vi "Insert Key Value Pair (Nested Boolean).vi"(7 "key":string[](array[string]), 8 "error in (no error)":errorcluster, 10 "JSON Data in":bool, 11 "JSON Object in":refnum<class "JSON Helper.lvclass">) -> (0 "error out":errorcluster, 1 "replaced":bool, 3 "JSON Object Out":refnum<class "JSON Helper.lvclass">)   [LabVIEW 2016, in "JSON Helper.lvclass"]
uses:
  JSON Helper/JSON Helper.lvclass
  JSON Datatype/JSON Null.lvclass
  JSON Array/Replace Array Subset (Single).vi
  JSON Helper/To More Specific Type (Object).vi
  JSON Helper/To More Specific Type (Array).vi
  JSON Boolean/New JSON Boolean.vi
  Insert Key Value Pair (Single String).vi
  JSON Array/JSON Array.lvclass
  JSON Object.lvclass
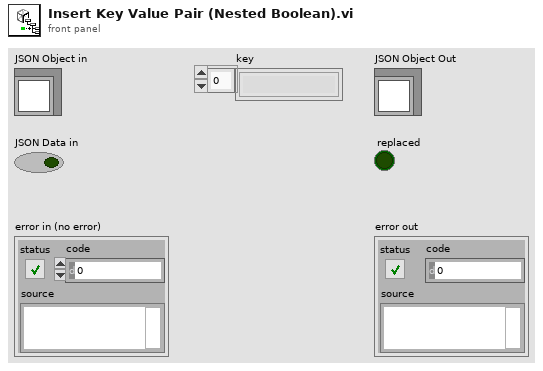
[diagram p1: front panel]
types:
  T1 = typedef "JSON Helper.lvclass/JSON Types.ctl" = enum16{"String", "Numeric", "Boolean", "NULL", "Object", "Array"}
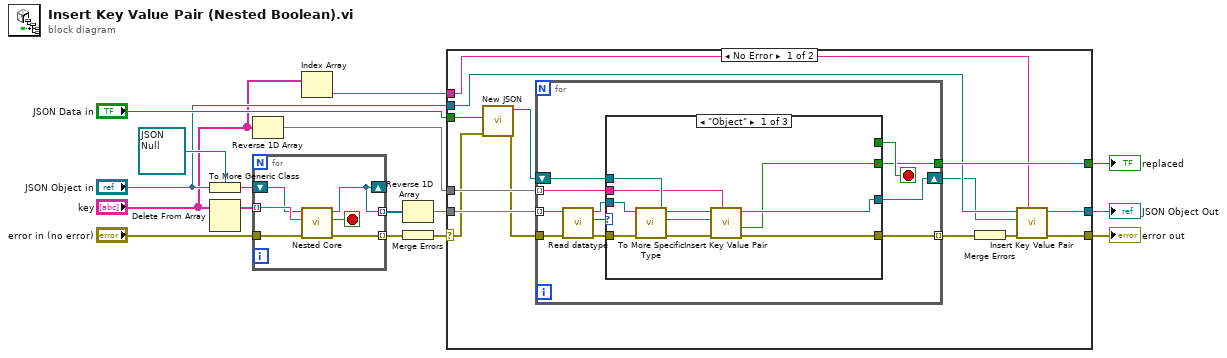
[diagram p0: block diagram]
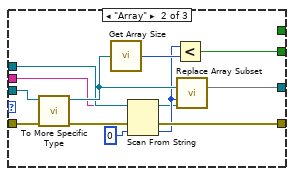
[diagram p2: hidden frame]
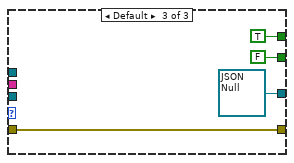
[diagram p3: hidden frame]
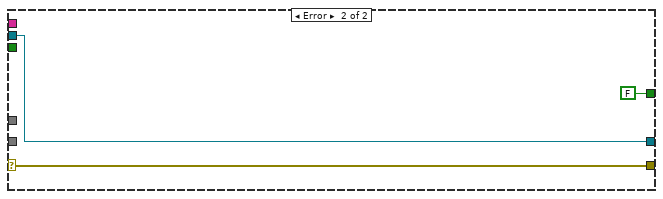
[diagram p4: hidden frame]
diagram:
  n1 = To More Generic Class(target class=refnum<class "JSON Null.lvclass"> refnum, reference="JSON Object in") -> (generic class reference=w8:refnum<class "JSON Null.lvclass">)
  n2 = Delete From Array(array="key") -> (array with subset deleted=w12:string[])  [unwired: 2 in, 1 out]
  n3 = Reverse 1D Array(array="key") -> (reversed array=w13:string[])
  n4 = for {
    tunnel: w12 -> [w22] mode=indexing
    shift-right: [w17] -> _
    shift-left: w8 -> [w21]
    tunnel: "error in (no error)" -> [w20]
    tunnel: [w19] -> w9 mode=indexing
    tunnel: [w17] -> w10 mode=indexing
    stop <- w18 stop-if-true
    n5 = call "Nested Core.vi"("error in (no error)"=w20, "key"=w22, "JSON in"=w21) -> ("error out"=w19:errorcluster, "stop?"=w18:bool, "JSON out"=w17:refnum<class "JSON Helper.lvclass">)  [unwired: 6 in]
  }
  n6 = Index Array(array="key") -> (element=w1:string)  [unwired: 1 in]
  n7 = Reverse 1D Array(array=w10) -> (reversed array=w14:refnum<class "JSON Helper.lvclass">[])
  n8 = Merge Errors(w9) -> (w11:errorcluster)
  n9 = case shown="No Error" w11 {
    selector: w11 -> [w24 w73]
    tunnel: [w36 FALSE ("replaced")] -> w16
    tunnel: "JSON Data in" -> [w26 _]
    tunnel: w14 -> [w35 _]
    tunnel: w13 -> [w34 _]
    tunnel: [w30 w75] -> w4
    tunnel: "JSON Object in" -> [w32 w75]
    tunnel: [w28 w73] -> w3
    tunnel: w1 -> [w27 _]
    frame No Error {
      n10 = call-poly "New JSON.vi"("error in (no error)"=w24, "value"=w26) -> ("error out"=w23:errorcluster, "JSON Boolean out"=w25:refnum<class "JSON Helper.lvclass">)  [unwired: 8 in]
      n11 = for {
        tunnel: w34 -> [w39] mode=indexing
        tunnel: w23 -> [w45]
        tunnel: [w44] -> w33 mode=indexing
        tunnel: [w41] -> w36
        tunnel: w35 -> [w40] mode=indexing
        shift-right: [w38] -> w31
        shift-left: w25 -> [w37]
        stop <- w42 stop-if-true
        n12 = call "Read datatype.vi"("error in (no error)"=w45, "JSON Datatype in"=w40) -> ("error out"=w43:errorcluster, "datatype"=w46:T1, "JSON Datatype out"=w47:refnum<class "JSON Helper.lvclass">)  [unwired: 7 in]
        n13 = case shown="\"Object\"" w46 {
          tunnel: w39 -> [w48 w57 _]
          tunnel: [w50 w59 refnum<class "JSON Null.lvclass"> refnum ("JSON Data")] -> w38
          tunnel: w47 -> [w55 w68 _]
          tunnel: [w52 w64 w70] -> w44
          tunnel: w43 -> [w54 w66 w70]
          tunnel: [_ _ TRUE] -> w42
          tunnel: [w49 w60 FALSE] -> w41
          tunnel: w37 -> [w51 w58 _]
          frame "Object" {
            n14 = call-poly "To More Specific Type.vi"("error in (no error)"=w54, "JSON Datatype in"=w55) -> ("error out"=w53:errorcluster, "JSON Datatype out"=w56:refnum<class "JSON Object.lvclass">)  [unwired: 8 in]
            n15 = call-poly "Insert Key Value Pair.vi"("key"=w48, "error in (no error)"=w53, "value"=w51, "JSON Object in"=w56) -> ("error out"=w52:errorcluster, "replaced"=w49:bool, "JSON Object out"=w50:refnum<class "JSON Helper.lvclass">)  [unwired: 5 in]
          }
          frame "Array" {
            n16 = call-poly "To More Specific Type.vi"("error in (no error)"=w66, "JSON Datatype in"=w68) -> ("error out"=w65:errorcluster, "JSON Datatype out"=w63:refnum<class "JSON Array.lvclass">)  [unwired: 8 in]
            n17 = call "Get Array Size.vi"("JSON Array in"=w63) -> ("size(s)"=w62:i32)
            n18 = Scan From String(input string=w57, error in=w65, default 1=0 ("index")) -> (error out=w64:errorcluster, output 1=w61:i32)  [unwired: 2 in, 2 out]
            n19 = Less?(x=w61, y=w62) -> (x < y?=w60:bool)
            n20 = call-poly "Replace Array Subset.vi"(5:w63, "new element/subarray"=w61, "error in"=w58) -> (6:w59)  [unwired: 10 in, 2 out]
          }
          frame Default {
          }
        }
      }
      n21 = Merge Errors(w33) -> (w29:errorcluster)
      n22 = call-poly "Insert Key Value Pair.vi"("key"=w27, "error in (no error)"=w29, "value"=w31, "JSON Object in"=w32) -> ("error out"=w28:errorcluster, "JSON Object out"=w30:refnum<class "JSON Helper.lvclass">)  [unwired: 5 in, 1 out]
    }
    frame Error {
    }
  }
  "replaced" <- w16
  "error out" <- w3
  "JSON Object Out" <- w4
